vi "Plugin.Get Debug Flags.vi"(11 "Plugin in":refnum<class "Plugin.lvclass">) -> (2 "Debug Flags":refnum<class "Debug Flags.lvclass">, 3 "Plugin out":refnum<class "Plugin.lvclass">)   [LabVIEW 2017, in "DSF Core.lvlib" / "Plugin.lvclass"]
uses:
  Plugin.lvclass
  Debug/Debug Flags/Debug Flags.lvclass
  Plugin.lvclass/Plugin.ctl
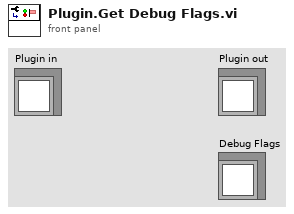
[diagram p1: front panel]
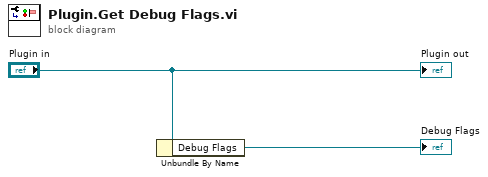
[diagram p0: block diagram]
diagram:
  n1 = Unbundle By Name("Plugin in") -> ("Debug Flags"=→"Debug Flags":refnum<class "Debug Flags.lvclass">)
  "Plugin out" <- "Plugin in"
